vi "LeCroy.Open Session.vi"(8 "Error In":errorcluster, 11 "VISA resource name":refnum<visa-resource-name>) -> (0 "Error Out":errorcluster, 3 "LeCroy.Session out":T1)   [LabVIEW 2018]
uses:
  typedefs/LeCroy.Session.ctl
  Driver/lecroy_wave_series/LeCroy Wave Series/LeCroy Wave Series.lvlib
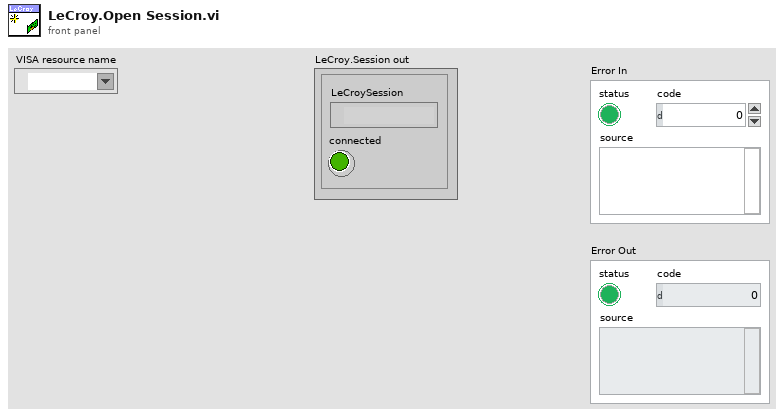
[diagram p1: front panel]
types:
  T1 = typedef "LeCroy.Session.ctl" = cluster{"LeCroySession":refnum<visa-resource-name>, "connected":bool}
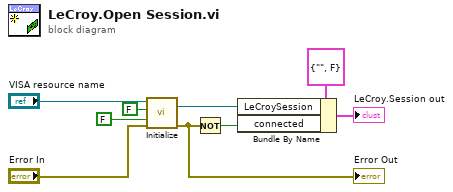
[diagram p0: block diagram]
diagram:
  n1 = call "Initialize.vi"("error in (no error)"="Error In", "Reset? (T: Yes)"=FALSE, "ID Query? (T: Yes)"=FALSE, "VISA resource name"="VISA resource name") -> ("error out"=w3:errorcluster, "VISA resource name out"=w5:refnum<visa-resource-name>)  [unwired: 6 in]
  "Error Out" <- w3
  n2 = Not(x=w3) -> (.not. x?=w4:bool)
  n3 = Bundle By Name(cluster=T1 {"LeCroySession"="", "connected"=FALSE} ("LeCroy.Session"), "LeCroySession"=w5, "connected"=w4) -> (→"LeCroy.Session out":T1)
